vi "Character LCD Class.vi"() -> ()   [LabVIEW 2020]
uses:
  CTI-Peripheral/Character LCD/Char LCD.lvclass
panel:
  in  "Char LCD":refnum<class "Char LCD.lvclass">
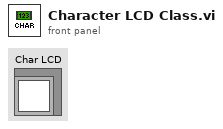
[diagram p1: front panel]
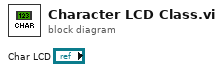
[diagram p0: block diagram]
diagram:
